vi "Borrowed Lockin SR830.vi"(8 "error in (no error)":errorcluster, 10 "Is SR830? (T)":bool=TRUE, 11 "Lockin SR830 in":refnum<class "Lockin SR830.lvclass">) -> (0 "error out":errorcluster, 3 "Lockin SR830 out":refnum<class "Lockin SR830.lvclass">)   [LabVIEW 2009, in "Lockin SR830.lvclass"]
uses:
  Lockin SR830.lvclass
  Lockin SR830.lvclass/Lockin SR830.ctl
  Global/GPIB Numbers.vi
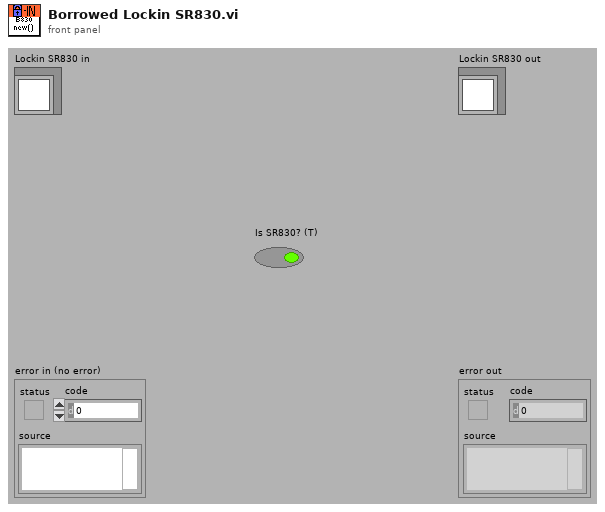
[diagram p1: front panel]
types:
  T1 = typedef "GPIB Type Def.ctl" = cluster{"Name":string, "bus":dbl, "GPIB":dbl, "GPIB as string":string, "byte":i32, "VISA Resource Name":refnum<visa-resource-name>}
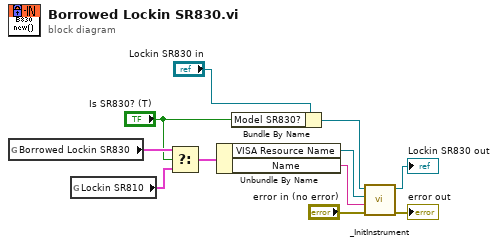
[diagram p0: block diagram]
diagram:
  n1 = global read "GPIB Numbers.vi" "Borrowed Lockin SR830"() -> (w4:T1)
  n2 = global read "GPIB Numbers.vi" "Lockin SR810"() -> (w5:T1)
  n3 = Select(t=w4, s="Is SR830? (T)", f=w5) -> (s? t:f=w3:T1)
  n4 = Unbundle By Name(w3) -> ("VISA Resource Name"=w1:refnum<visa-resource-name>, "Name"=w6:string)
  n5 = Bundle By Name(cluster="Lockin SR830 in", "Model SR830?"="Is SR830? (T)") -> (w10:refnum<class "Lockin SR830.lvclass">)
  n6 = call-dynamic "_InitInstrument.vi"("error in (no error)"="error in (no error)", "Name"=w6, "VISA Resource Name"=w1, "Instrument in"=w10) -> ("error out"=→"error out":errorcluster, "Instrument out"=→"Lockin SR830 out":refnum<class "Lockin SR830.lvclass">)  [unwired: 2 in, 4 out]
